vi "Update Digital Pattern FPGA Resources.vi"(8 "error in (no error)":errorcluster, 11 "Page Data in":T1={"SysExp Event"=refnum, "Init done"=FALSE, "Node Ptr"=18446744073709551615, "Ctrl Refs"={"Header"=refnum, "Pattern Plot"=refnum, "Zoom"=refnum, "Select Pattern"=refnum, "Add List"=refnum, "Remove List"=refnum, "Pattern Name"=refnum, "remove_add"=refnum, "remove_remove"=refnum, "add_remove"=refnum, "base_Length"=refnum, "base_teeth"=refnum, "base_Toothwidth"=refnum, "base_Offset"=refnum, "add_Tooth"=refnum, "add_Width"=refnum, "add_Offset"=refnum, "remove_Tooth"=refnum, "remove_Edge"=refnum, "Chart_Position"=refnum, "Chart_Tooth"=refnum, "Chart_Offset"=refnum, "add_add"=refnum, "pattern_remove"=refnum, "pattern_add"=refnum, "FPGA Resource"=refnum}, "SE ref"=refnum, "Patterns"=[], "Sel patterns"=[], "rotations"=0, "Need save"=FALSE, "Rem List"=0, "Add List"=0, "FPGA Resources"=[]} {"Node Ptr" format="%.0x"}) -> (0 "error out":errorcluster)   [LabVIEW 2017, in "Engine Simulation Toolkit System Explorer.lvlib"]
uses:
  Engine Simulation Toolkit System Explorer.lvlib
  Digital Patterns Page Data.ctl
  <vilib>/NI Veristand/Custom Device API/Custom Device Item Ref.ctl
  Digital Pattern.ctl
  Digital Pattern Base.ctl
  Digital Pattern Remove Edge.ctl
  Digital Pattern Add Pulse.ctl
  <vilib>/NI Veristand/Custom Device API/Custom Device API.lvlib
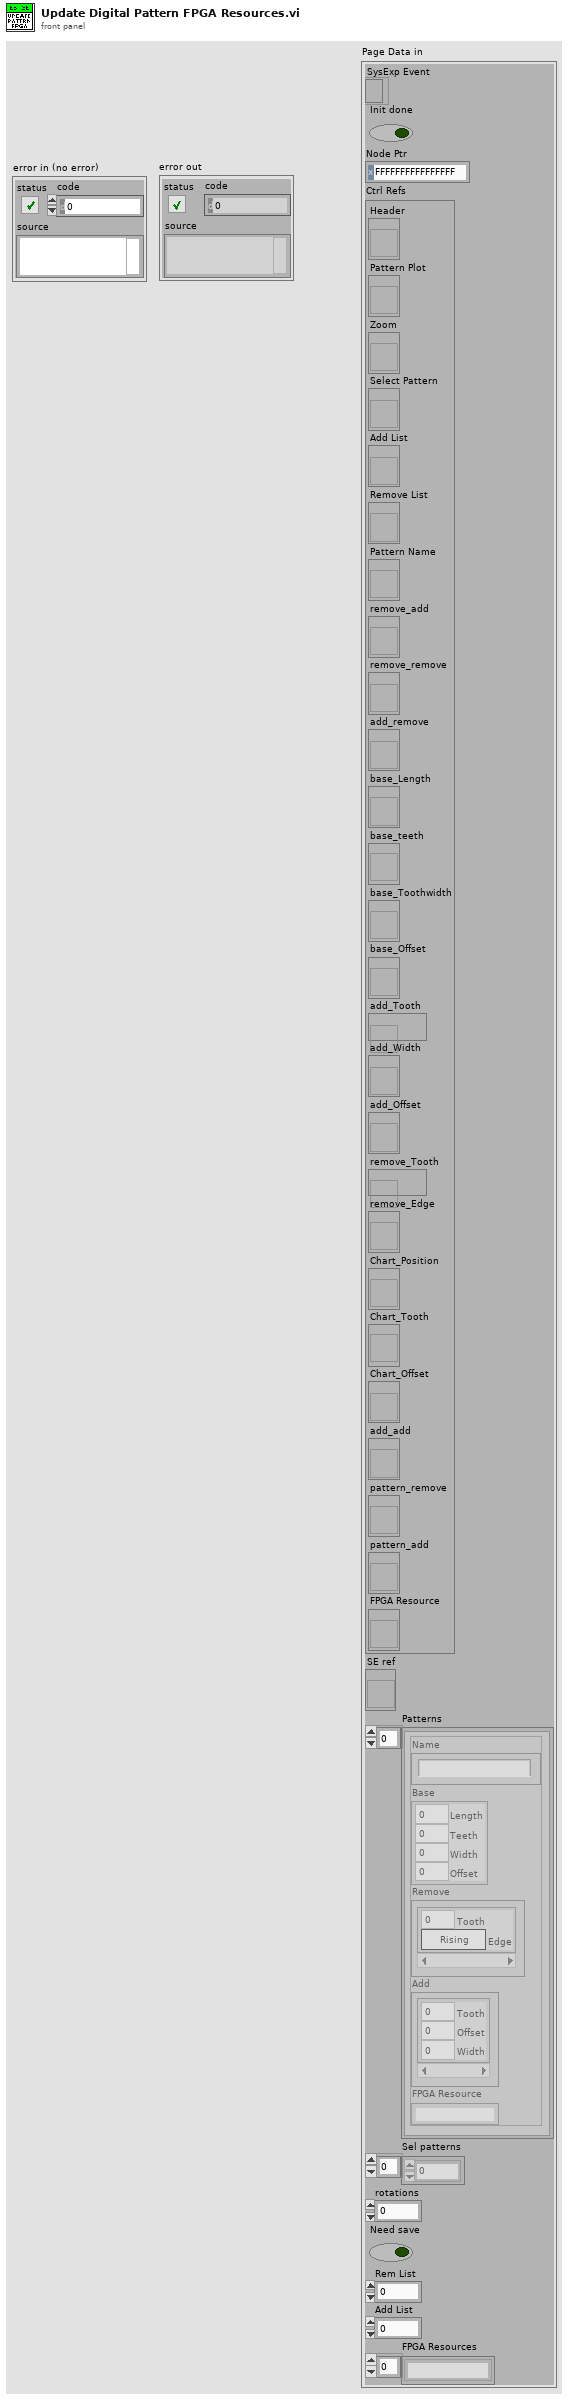
[diagram p1: front panel]
types:
  T1 = typedef "Engine Simulation Toolkit System Explorer.lvlib/Digital Patterns Page Data.ctl" = cluster{"SysExp Event":refnum<event-registration>, "Init done":bool, "Node Ptr":T2, "Ctrl Refs":cluster{"Header":refnum<vi>, "Pattern Plot":refnum<vi>, "Zoom":refnum<vi>, "Select Pattern":refnum<vi>, "Add List":refnum<vi>, "Remove List":refnum<vi>, "Pattern Name":refnum<vi>, "remove_add":refnum<vi>, "remove_remove":refnum<vi>, "add_remove":refnum<vi>, "base_Length":refnum<vi>, "base_teeth":refnum<vi>, "base_Toothwidth":refnum<vi>, "base_Offset":refnum<vi>, "add_Tooth":refnum<vi>, "add_Width":refnum<vi>, "add_Offset":refnum<vi>, "remove_Tooth":refnum<vi>, "remove_Edge":refnum<vi>, "Chart_Position":refnum<vi>, "Chart_Tooth":refnum<vi>, "Chart_Offset":refnum<vi>, "add_add":refnum<vi>, "pattern_remove":refnum<vi>, "pattern_add":refnum<vi>, "FPGA Resource":refnum<vi>}, "SE ref":refnum<vi>, "Patterns":T3[], "Sel patterns":i32[], "rotations":u16, "Need save":bool, "Rem List":i32, "Add List":i32, "FPGA Resources":string[]}
  T2 = typedef "Custom Device API.lvlib/Custom Device Item Ref.ctl" = u64
  T3 = typedef "Engine Simulation Toolkit System Explorer.lvlib/Digital Pattern.ctl" = cluster{"Name":string, "Base":T4, "Remove":T5[], "Add":T6[], "FPGA Resource":string}
  T4 = typedef "Engine Simulation Toolkit System Explorer.lvlib/Digital Pattern Base.ctl" = cluster{"Length":dbl, "Teeth":u16, "Width":dbl, "Offset":dbl}
  T5 = typedef "Engine Simulation Toolkit System Explorer.lvlib/Digital Pattern Remove Edge.ctl" = cluster{"Tooth":u16, "Edge":bool}
  T6 = typedef "Engine Simulation Toolkit System Explorer.lvlib/Digital Pattern Add Pulse.ctl" = cluster{"Tooth":u16, "Offset":dbl, "Width":dbl}
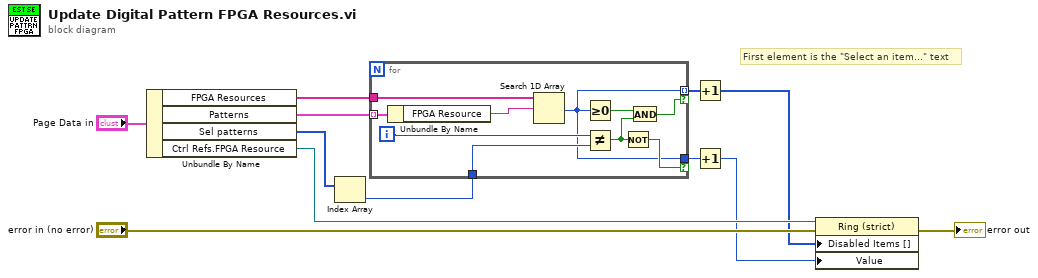
[diagram p0: block diagram]
diagram:
  # "First element is the \"Select an item...\" text"
  n1 = Unbundle By Name("Page Data in") -> ("FPGA Resources"=w7:string[], "Patterns"=w11:T3[], "Sel patterns"=w12:i32[], "Ctrl Refs.FPGA Resource"=w9:refnum<vi>)
  n2 = Index Array(array=w12) -> (element=w5:i32)  [unwired: 1 in]
  n3 = for {
    tunnel: w11 -> [w22] mode=indexing
    tunnel: w7 -> [w21]
    tunnel: [w13] -> w6 mode=indexing if=w19
    tunnel: w5 -> [w17]
    tunnel: [w13] -> w2 if=w14
    i -> [w18]
    n4 = Unbundle By Name(w22) -> ("FPGA Resource"=w16:string)
    n5 = Search 1D Array(1D array=w21, element=w16) -> (index of element=w13:i32)  [unwired: 1 in]
    n6 = Greater Or Equal To 0?(x=w13) -> (x >= 0?=w20:bool)
    n7 = Not Equal?(x=w18, y=w17) -> (x != y?=w15:bool)
    n8 = Not(x=w15) -> (.not. x?=w14:bool)
    n9 = And(x=w20, y=w15) -> (x .and. y?=w19:bool)
  }
  n10 = Increment(x=w6) -> (x+1=w4:i32[])
  n11 = Increment(x=w2) -> (x+1=w1:i32)
  n12 = property class="Ring (strict)"(reference=w9, error in="error in (no error)", "Disabled Items []"=w4, "Value"=w1) -> (error out=→"error out":errorcluster)  [unwired: 1 out]
